vi "Line Detector Smooth.vi"(8 "error in (no error)":errorcluster, 9 "Frequency step":dbl, 10 "Signal":cdb[](array[numeric]), 11 "Line Detector Configuration":T1={"Peak width guess"=500.0, "Background removal"=enum."High-pass", "Smoothing"=enum."Low-pass", "Smooth window"=200.0, "Relative threshold"=0.2, "Finder algorithm"=enum."Wavelet", "Bgd window"=50000.0, "Spectrum recorder module name"="Spectrum Recorder", "Fit window"=1000.0, "Initial fit guess"=enum."Peak finder", "...with header "="", "Create rusin.dat"=FALSE, "Follow\npeaks"=FALSE} {"Fit window" format="%#_6pHz"; "Bgd window" format="%#_6pHz"; "Smooth window" format="%#_6pHz"; "Peak width guess" format="%#_6pHz"}) -> (0 "error out":errorcluster, 2 "Signal out":cdb[](array[numeric]))   [LabVIEW 2016]
uses:
  LabActor/Post-Processors/Line Detector/Line Detector Configuration.ctl
  <vilib>/addons/Wavelet Analysis/application.llb/WA Denoise (DWT Real Array).vi
  <vilib>/addons/Wavelet Analysis/application.llb/WA Detrend (Array).vi
  <vilib>/addons/_Advanced Signal Processing/NI_AdvSigProcWA.lvlib
panel:
  # "Peak finder config"
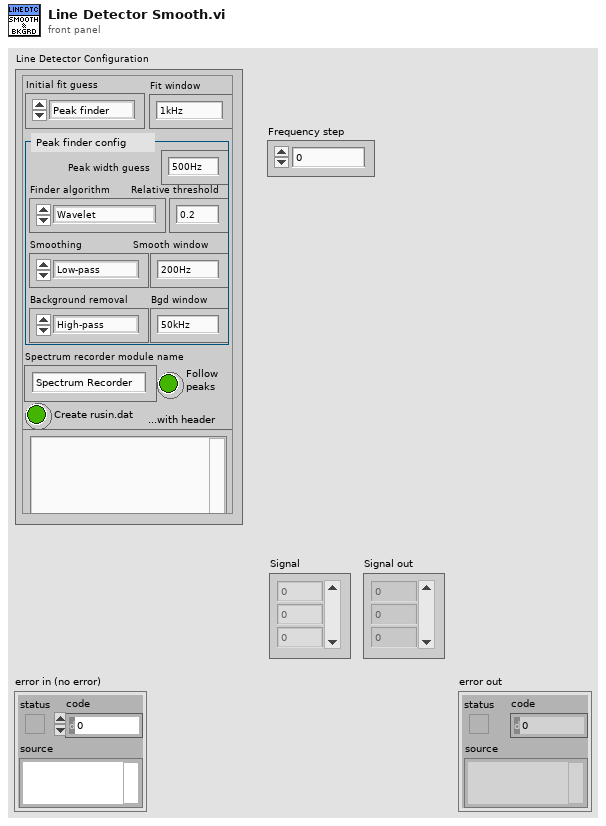
[diagram p1: front panel]
types:
  T1 = typedef "Line Detector Configuration.ctl" = cluster{"Peak width guess":dbl, "Background removal":enum16{"NONE", "High-pass", "Detrend"}, "Smoothing":enum16{"NONE", "Low-pass", "Denoise"}, "Smooth window":dbl, "Relative threshold":dbl, "Finder algorithm":enum16{"Basic", "Wavelet", "Wavelet+detrend"}, "Bgd window":dbl, "Spectrum recorder module name":string, "Fit window":dbl, "Initial fit guess":enum16{"Peak finder", "Last fit"}, "...with header ":string, "Create rusin.dat":bool, "Follow\npeaks":bool}
  T2 = enum16{"Lowpass", "Highpass", "Bandpass", "Bandstop"}
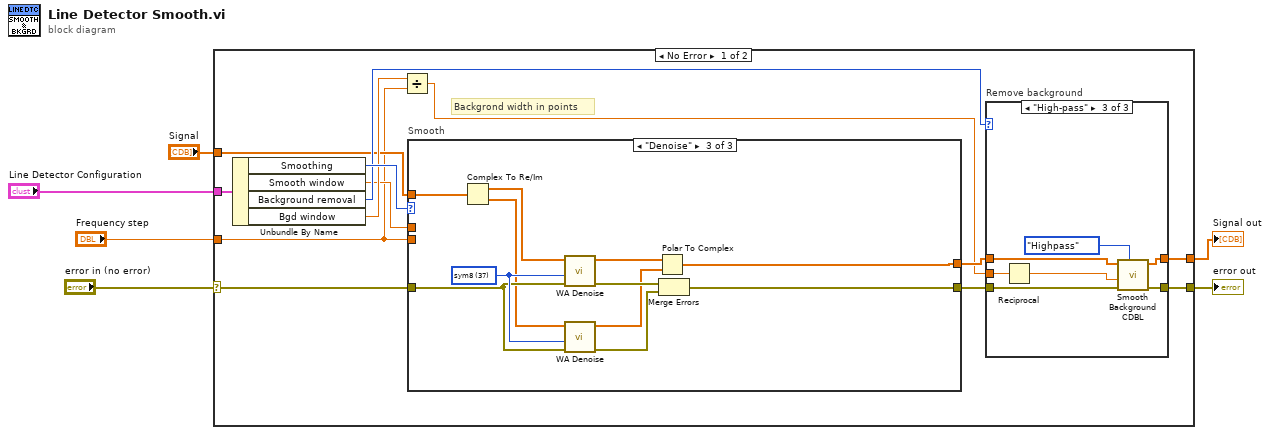
[diagram p0: block diagram]
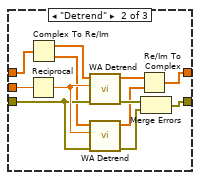
[diagram p3: hidden frame]
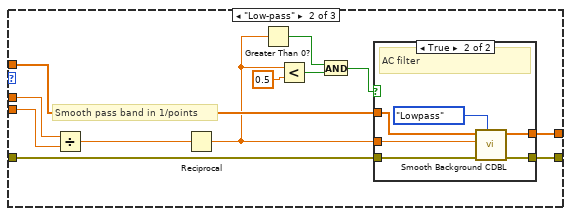
[diagram p5: hidden frame]
diagram:
  n1 = case shown="No Error" "error in (no error)" {
    selector: "error in (no error)" -> [w18 w75]
    tunnel: "Line Detector Configuration" -> [w19 _]
    tunnel: [w8 w75] -> w4
    tunnel: "Signal" -> [w10 w74]
    tunnel: "Frequency step" -> [w9 _]
    tunnel: [w7 w74] -> w1
    frame No Error {
      # "Backgrond width in points"
      n2 = Unbundle By Name(w19) -> ("Smoothing"=w17:enum16{"NONE", "Low-pass", "Denoise"}, "Smooth window"=w11:dbl, "Background removal"=w16:enum16{"NONE", "High-pass", "Detrend"}, "Bgd window"=w13:dbl)
      n3 = Divide(x=w13, y=w9) -> (x/y=w12:dbl)
      n4 = case "Smooth" shown="\"Denoise\"" w17 {
        tunnel: w10 -> [w42 w54 w68]
        tunnel: [w42 w53 w63] -> w15
        tunnel: w18 -> [w41 w51 w72]
        tunnel: [w41 w52 w69] -> w14
        tunnel: w11 -> [_ w45 _]
        tunnel: w9 -> [_ w44 _]
        frame "NONE", Default {
        }
        frame "Low-pass" {
          # "Smooth pass band in 1/points"
          n5 = Divide(x=w45, y=w44) -> (x/y=w43:dbl)
          n6 = Reciprocal(x=w43) -> (1/x=w49:dbl)
          n7 = Greater Than 0?(x=w49) -> (x > 0?=w48:bool)
          n8 = Less?(x=w49, y=0.5) -> (x < y?=w47:bool)
          n9 = And(x=w48, y=w47) -> (x .and. y?=w46:bool)
          n10 = case shown="True" w46 {
            tunnel: w54 -> [w56 w61]
            tunnel: [w56 w57] -> w53
            tunnel: [w55 w60] -> w52
            tunnel: w51 -> [w55 w59]
            tunnel: w49 -> [_ w58]
            frame False {
              # "Bypass if band too narrow"
            }
            frame True {
              # "AC filter"
              n11 = call "Smooth Background CDBL.vi"("Type"=T2."Lowpass", "Error In"=w59, "LP  F"=w58, "Data"=w61) -> ("Error Out"=w60:errorcluster, "Data out"=w57:cdb[])  [unwired: 6 in]
            }
          }
        }
        frame "Denoise" {
          w73 = u16 37 items=["db02"=0, "db03"=1, "db04"=2, "db05"=3, "db06"=4, "db07"=5, "db08"=6, "db09"=7, "db10"=8, "db11"=9, "db12"=10, "db13"=11, "db14"=12, "Haar"=13, "bior1_3"=14, "bior1_5"=15, "bior2_2"=16, "bior2_4"=17, "bior2_6"=18, "bior2_8"=19, "bior3_1"=20, "bior3_3"=21, "bior3_5"=22, "bior3_7"=23, "bior3_9"=24, "bior4_4 (FBI)"=25, "bior5_5"=38, "bior6_8"=39, "coif1"=26, "coif2"=27, "coif3"=28, "coif4"=29, "coif5"=30, "sym2"=31, "sym3"=32, "sym4"=33, "sym5"=34, "sym6"=35, "sym7"=36, "sym8"=37] ("wavelet")
          n12 = Complex To Re/Im(x + iy=w68) -> (x=w67:dbl[], y=w66:dbl[])
          n13 = call-poly <vilib>:"WA Denoise.vi"("error in (no error)"=w72, "wavelet"=w73, "signal"=w67) -> ("error out"=w71:errorcluster, "denoised signal"=w64:dbl[])  [unwired: 7 in]
          n14 = call-poly <vilib>:"WA Denoise.vi"("error in (no error)"=w72, "wavelet"=w73, "signal"=w66) -> ("error out"=w70:errorcluster, "denoised signal"=w65:dbl[])  [unwired: 7 in]
          n15 = Polar To Complex(1:w65, 2:w64) -> (0:w63:cdb[])
          n16 = Merge Errors(w71, w70) -> (w69:errorcluster)
        }
      }
      n17 = case "Remove background" shown="\"High-pass\"" w16 {
        tunnel: w15 -> [w21 w31 w38]
        tunnel: [w21 w22 w40] -> w7
        tunnel: w12 -> [_ w30 w37]
        tunnel: w14 -> [w20 w27 w36]
        tunnel: [w20 w28 w35] -> w8
        frame "NONE", Default {
        }
        frame "Detrend" {
          n18 = Reciprocal(x=w30) -> (1/x=w29:dbl)
          n19 = Complex To Re/Im(x + iy=w31) -> (x=w26:dbl[], y=w25:dbl[])
          n20 = call-poly <vilib>:"WA Detrend.vi"("error in (no error)"=w27, "threshold frequency"=w29, "signal"=w26) -> ("error out"=w32:errorcluster, "detrended signal"=w23:dbl[])  [unwired: 6 in, 1 out]
          n21 = call-poly <vilib>:"WA Detrend.vi"("error in (no error)"=w27, "threshold frequency"=w29, "signal"=w25) -> ("error out"=w33:errorcluster, "detrended signal"=w24:dbl[])  [unwired: 6 in, 1 out]
          n22 = Re/Im To Complex(1:w24, 2:w23) -> (0:w22:cdb[])
          n23 = Merge Errors(w32, w33) -> (w28:errorcluster)
        }
        frame "High-pass" {
          n24 = Reciprocal(x=w37) -> (1/x=w34:dbl)
          n25 = call "Smooth Background CDBL.vi"("Type"=T2."Highpass", "Error In"=w36, "HP F"=w34, "Data"=w38) -> ("Error Out"=w35:errorcluster, "Data out"=w40:cdb[])  [unwired: 6 in]
        }
      }
    }
    frame Error {
    }
  }
  "error out" <- w4
  "Signal out" <- w1
